vi "Configure Auto Load Compensation.vi"(6 "channel":i32=1 min=1 max=4, 8 "error in (no error)":errorcluster, 10 "auto load compensation":bool, 11 "VISA resource name":refnum<visa-resource-name>) -> (0 "error out":errorcluster, 3 "VISA resource name out":refnum<visa-resource-name>)   [LabVIEW 2019, in "Pulse Rider PG-1000.lvlib"]
doc: "Set the automatic calculation of the load impedance for the selected output channel. If the load compensation is set to ON, the value set through the command Load Impedence will be ignored.\n \nIMPORTANT NOTE: you can send this command only when the instrument is in stopped state.\n\nchannel: the output channel int from 1 to 4"
uses:
  <instrlib>/Pulse Rider PG-1000/Pulse Rider PG-1000.lvlib
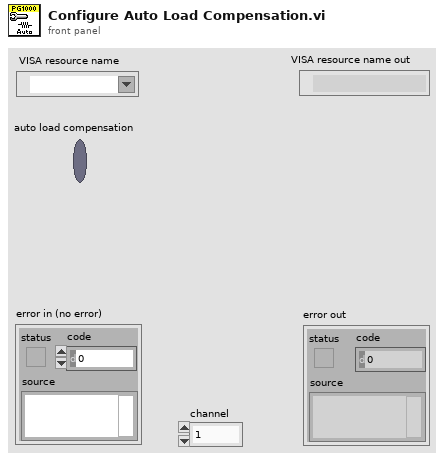
[diagram p1: front panel]
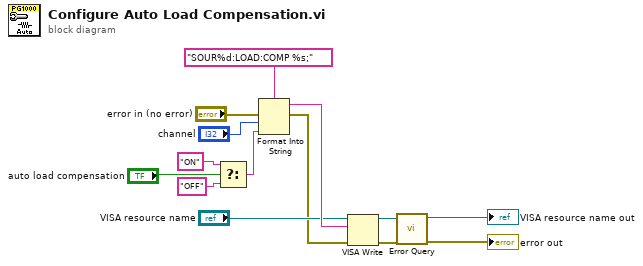
[diagram p0: block diagram]
diagram:
  n1 = Select(t="ON", s="auto load compensation", f="OFF") -> (s? t:f=w3:string)
  n2 = Format Into String(format string="SOUR%d:LOAD:COMP %s;", error in="error in (no error)", "channel", w3) -> (resulting string=w11:string, error out=w1:errorcluster)  [unwired: 1 in]
  n3 = VISA Write(VISA resource name="VISA resource name", write buffer=w11, error in (no error)=w1) -> (VISA resource name out=w14:refnum<visa-resource-name>, error out=w13:errorcluster)  [unwired: 1 out]
  n4 = call <instrlib>:"Error Query.vi"("error in (no error)"=w13, "VISA resource name"=w14) -> ("error out"=→"error out":errorcluster, "VISA resource name out"=→"VISA resource name out":refnum<visa-resource-name>)  [unwired: 6 in, 2 out]
